vi "Instrument Configure RF.vi"(0 "RFSG Session In":refnum<k15>, 5 "SG Configuration":T1={"Reference Clock Source"="OnboardClock", "Carrier Frequency (Hz)"=1000000000.0, "DUT Average Input Power (dBm)"=-20.0, "External Attenuation (dB)"=0.0, "Marker 0 Export Terminal"="PXI_Trig0", "Share LO  SG->SA"=FALSE} {"Carrier Frequency (Hz)" format="%#_6p"}, 11 "error in (no error)":errorcluster) -> (4 "RFSG Session Out":refnum<k15>, 15 "error out":errorcluster)   [LabVIEW 2018, in "SG.lvlib"]
doc: "All unwired terminals will be ignored; only valid values will be set"
uses:
  SG.lvlib
  Typedefs/Instrument Configuration.ctl
  <instrlib>/niRFSG/niRFSG.llb/niRFSG Ref Clock Sources.ctl
  <instrlib>/niRFSG/niRFSG.llb/niRFSG Trigger Terminals.ctl
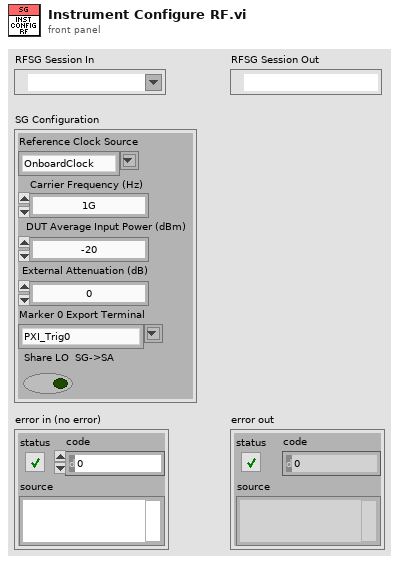
[diagram p1: front panel]
types:
  T1 = typedef "SG.lvlib/Instrument Configuration.ctl" = cluster{"Reference Clock Source":T2, "Carrier Frequency (Hz)":dbl, "DUT Average Input Power (dBm)":dbl, "External Attenuation (dB)":dbl, "Marker 0 Export Terminal":T3, "Share LO  SG->SA":bool}
  T2 = typedef "niRFSG Ref Clock Sources.ctl" = string
  T3 = typedef "niRFSG Trigger Terminals.ctl" = string
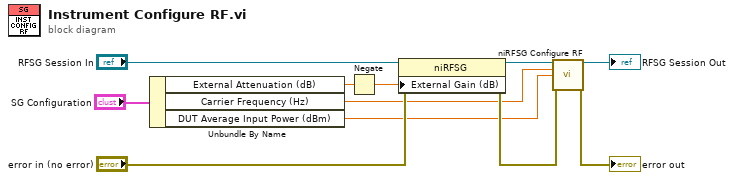
[diagram p0: block diagram]
diagram:
  n1 = Unbundle By Name("SG Configuration") -> ("External Attenuation (dB)"=w7:dbl, "Carrier Frequency (Hz)"=w3:dbl, "DUT Average Input Power (dBm)"=w2:dbl)
  n2 = Negate(x=w7) -> (-x=w1:dbl)
  n3 = property class="niRFSG"(reference="RFSG Session In", error in="error in (no error)", "External Gain (dB)"=w1) -> (reference out=w9:refnum<k15>, error out=w5:errorcluster)
  n4 = call <instrlib>:"niRFSG Configure RF.vi"("instrument handle"=w9, "frequency (Hz)"=w3, "power level (dBm)"=w2, "error in"=w5) -> ("instrument handle out"=→"RFSG Session Out":refnum<k15>, "error out"=→"error out":errorcluster)  [unwired: 10 in]
